vi "Create Mesh Grid (2D) (x,y arrays).vi"(10 "y domain":dbl[](array[numeric]), 11 "x domain":dbl[](array[numeric])) -> (0 "error":i32, 2 "Y":dbl[][](array[numeric]), 3 "X":dbl[][](array[numeric]))   [LabVIEW 2010, in "NI_Gmath.lvlib"]
doc: "Takes two <B>x domain</B> and <B>y domain</B> arrays and forms <B>X</B> and <B>Y</B> 2D arrays, which are typically used to evaluate and plot functions of two variables. You must manually select the polymorphic instance to use."
uses:
  NI_Gmath.lvlib
panel:
  # "Create Mesh Grid (2D)"
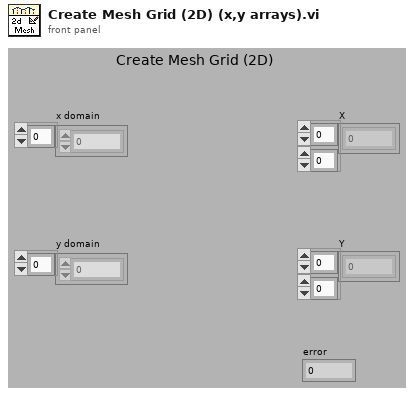
[diagram p1: front panel]
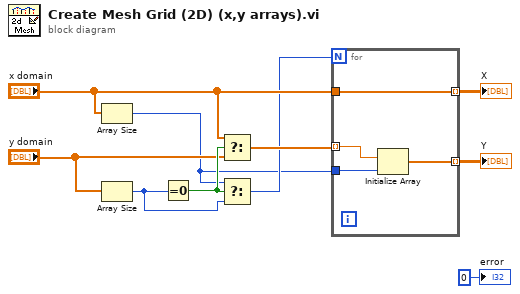
[diagram p0: block diagram]
diagram:
  n1 = Array Size(array="x domain") -> (size(s)=w2:i32)
  n2 = Array Size(array="y domain") -> (size(s)=w4:i32)
  n3 = Equal To 0?(x=w4) -> (x = 0?=w8:bool)
  n4 = Select(t="x domain", s=w8, f="y domain") -> (s? t:f=w6:dbl[])
  n5 = Select(t=w2, s=w8, f=w4) -> (s? t:f=w3:i32)
  n6 = for {
    N: w3 -> [_]
    tunnel: "x domain" -> [w14]
    tunnel: [w14] -> w10 mode=indexing
    tunnel: w6 -> [w13] mode=indexing
    tunnel: [w12] -> w9 mode=indexing
    tunnel: w2 -> [w11]
    n7 = Initialize Array(w13, w11) -> (w12:dbl[])
  }
  "X" <- w10
  "Y" <- w9
  "error" <- 0 ("error")
